vi "base path.vi"() -> (3 "base path":path)   [LabVIEW 2018]
uses:
  <vilib>/Utility/sysdir.llb/System Directory Type.ctl
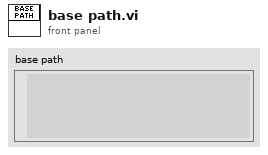
[diagram p1: front panel]
types:
  T1 = typedef "System Directory Type.ctl" = i32
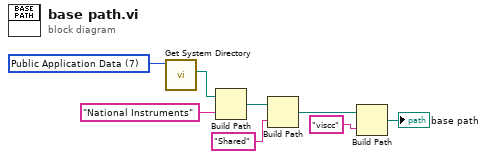
[diagram p0: block diagram]
diagram:
  w8 = T1 7 items=["User Home"=0, "User Desktop"=1, "User Documents"=2, "User Application Data"=3, "User Preferences"=4, "User Temporary"=5, "Public Documents"=6, "Public Application Data"=7, "Public Preferences"=8, "Public Cache"=13, "System Core Libraries"=9, "System Installed Libraries"=10, "Application Files"=11, "Boot Volume Root"=12] ("system directory type")
  n1 = call <vilib>:"Get System Directory.vi"("system directory type"=w8) -> ("system directory"=w1:path)  [unwired: 10 in]
  n2 = Build Path(base path=w1, name or relative path="National Instruments") -> (appended path=w5:path)
  n3 = Build Path(base path=w5, name or relative path="Shared") -> (appended path=w6:path)
  n4 = Build Path(base path=w6, name or relative path="viscc") -> (appended path=→"base path":path)
